vi "SetGraphParamsV2.vi"(7 "GraphRefArr":refnum<vi>[](array[refnum]), 8 "error in":errorcluster caption="entrée d'erreur (pas d'erreur)", 10 "CuurGrphCrvInd":i32[](array[numeric]), 11 "CurveSetupsIn":T1[](array[typedef])) -> (0 "error out":errorcluster caption="sortie d'erreur")   [LabVIEW 2010, in "Interface.lvclass"]
uses:
  Interface Class/Interface.lvclass
  Interface Class/CurveSetup.ctl
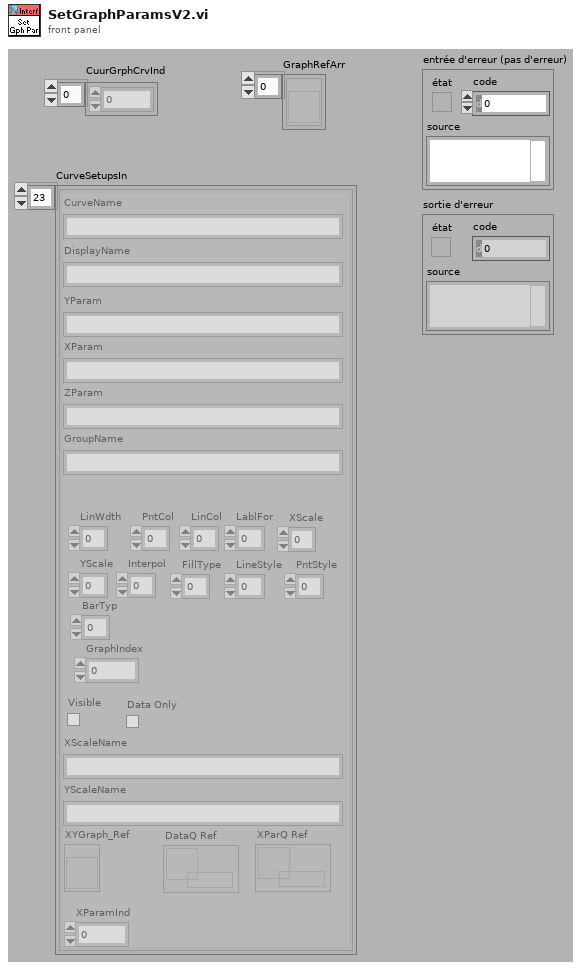
[diagram p1: front panel]
types:
  T1 = typedef "Interface.lvclass/CurveSetup.ctl" = cluster{"CurveName":string, "YParam":string, "XParam":string, "ZParam ":string, "GroupName":string, "LinWdth":u8, "PntCol":u32, "LinCol":u32, "LablFor":u8, "XScale":u32, "YScale":u32, "Interpol":u8, "DisplayName":string, "FillType":i16, "LineStyle":u8, "PntStyle":u8, "BarTyp":u8, "GraphIndex":i32, "Visible":bool, "XScaleName":string, "YScaleName":string, "XYGraph_Ref":refnum<vi>, "Data Only":bool, "DataQ Ref":refnum<queue>, "XParQ Ref":refnum<queue>, "XParamInd":i32}
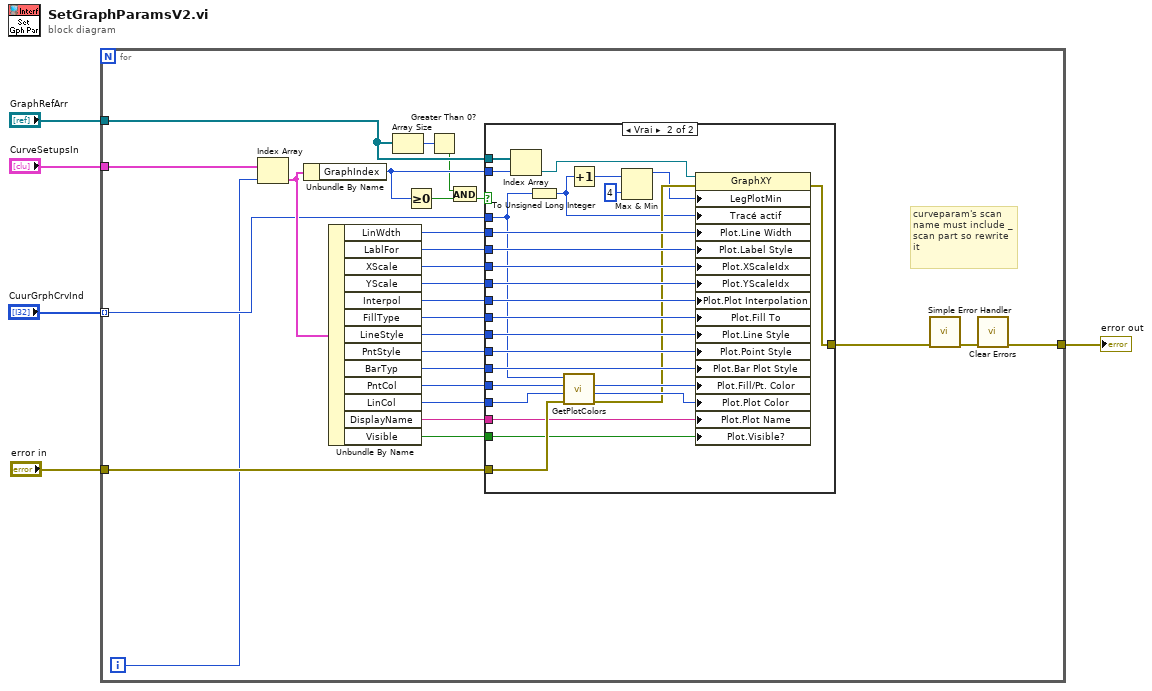
[diagram p0: block diagram]
diagram:
  n1 = for {
    tunnel: "GraphRefArr" -> [w32]
    tunnel: "error in" -> [w30]
    tunnel: [w29] -> w2
    tunnel: "CurveSetupsIn" -> [w31]
    tunnel: "CuurGrphCrvInd" -> [w7] mode=indexing
    i -> [w6]
    # "curveparam's scan name must include _scan part so rewrite it"
    n2 = Index Array(array=w31, index=w6) -> (element=w15:T1)
    n3 = Unbundle By Name(w15) -> ("GraphIndex"=w16:i32)
    n4 = Unbundle By Name(w15) -> ("LinWdth"=w28:u8, "LablFor"=w27:u8, "XScale"=w21:u32, "YScale"=w20:u32, "Interpol"=w26:u8, "FillType"=w25:i16, "LineStyle"=w24:u8, "PntStyle"=w23:u8, "BarTyp"=w22:u8, "PntCol"=w18:u32, "LinCol"=w17:u32, "DisplayName"=w8:string, "Visible"=w12:bool)
    n5 = Array Size(array=w32) -> (size(s)=w9:i32)
    n6 = Greater Or Equal To 0?(x=w16) -> (x >= 0?=w14:bool)
    n7 = Greater Than 0?(x=w9) -> (x > 0?=w10:bool)
    n8 = And(x=w10, y=w14) -> (x .and. y?=w11:bool)
    n9 = case shown="Vrai" w11 {
      tunnel: w28 -> [_ w59]
      tunnel: w27 -> [_ w58]
      tunnel: w26 -> [_ w57]
      tunnel: w25 -> [_ w56]
      tunnel: w24 -> [_ w55]
      tunnel: w23 -> [_ w54]
      tunnel: w22 -> [_ w53]
      tunnel: w21 -> [_ w52]
      tunnel: w20 -> [_ w51]
      tunnel: w32 -> [_ w49]
      tunnel: w16 -> [_ w48]
      tunnel: [w33 w47] -> w19
      tunnel: w18 -> [_ w46]
      tunnel: w17 -> [_ w45]
      tunnel: w30 -> [w33 w42]
      tunnel: w7 -> [_ w36]
      tunnel: w12 -> [_ w35]
      tunnel: w8 -> [_ w34]
      frame False {
        # "trying to graph on unavailable graph"
      }
      frame True {
        n10 = Index Array(array=w49, index=w48) -> (element=w50:refnum<vi>)
        n11 = To Unsigned Long Integer(number=w36) -> (unsigned 32bit integer=w39:u32)
        n12 = call "GetPlotColors.vi"("ErrorIn(No Error)"=w42, "Color2In"=w45, "Color1In"=w46, "ColorIndex"=w36) -> ("sortie d'erreur"=w41:errorcluster, "Color2Out"=w43:u32, "Color1Out"=w44:u32)  [unwired: 4 in, 1 out]
        n13 = Increment(x=w39) -> (x+1=w37:u32)
        n14 = Max & Min(x=w37, y=u32 4) -> (max(x,y)=w40:u32)  [unwired: 1 out]
        n15 = property class="GraphXY"(reference=w50, error in=w41, "LegPlotMin"=w40, "Tracé actif"=w39, "Plot.Line Width"=w59, "Plot.Label Style"=w58, "Plot.XScaleIdx"=w52, "Plot.YScaleIdx"=w51, "Plot.Plot Interpolation"=w57, "Plot.Fill To"=w56, "Plot.Line Style"=w55, "Plot.Point Style"=w54, "Plot.Bar Plot Style"=w53, "Plot.Fill/Pt. Color"=w44, "Plot.Plot Color"=w43, "Plot.Plot Name"=w34, "Plot.Visible?"=w35) -> (error out=w47:errorcluster)  [unwired: 1 out]
      }
    }
    n16 = call <vilib>:"Simple Error Handler.vi"("error in (no error)"=w19) -> ("error out"=w13:errorcluster)  [unwired: 4 in, 4 out]
    n17 = call <vilib>:"Clear Errors.vi"("error in (no error)"=w13) -> ("error out"=w29:errorcluster)  [unwired: 6 in]
  }
  "error out" <- w2
